vi "extract_value_from_string.vi"(8 "error in (no error)":errorcluster, 11 "Input string":string) -> (0 "error out":errorcluster, 2 "Value":dbl, 3 "Rest of string":string)   [LabVIEW 2016, in "Chemyx_Syringe_Pump_driver.lvlib"]
doc: "Converts the first number of an input string into a number and output the rest of the string."
uses:
  Chemyx_Syringe_Pump_driver.lvlib
panel:
  # "Converts the first number of an input string into a number and output the rest of the string."
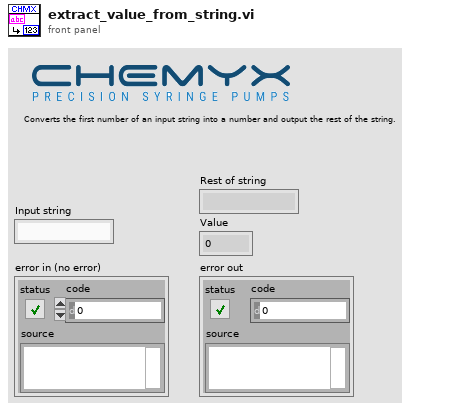
[diagram p1: front panel]
types:
  T1 = enum16{"Native", "Native Command Line", "UNIX", "Macintosh", "DOS"}
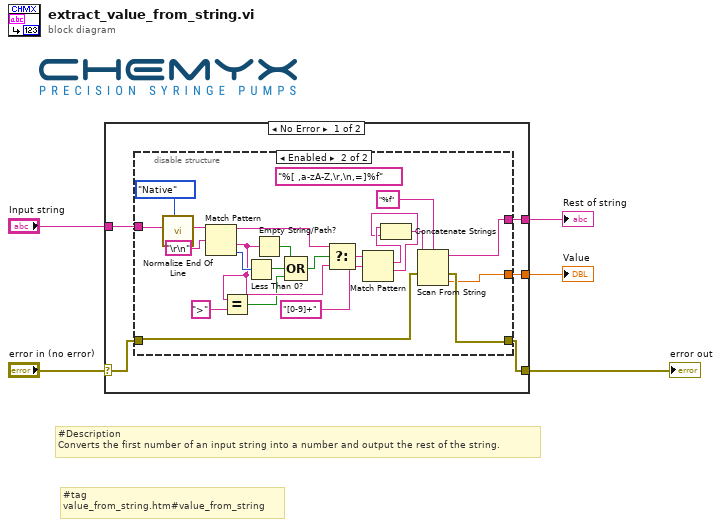
[diagram p0: block diagram]
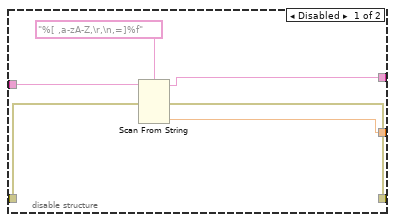
[diagram p2: hidden frame]
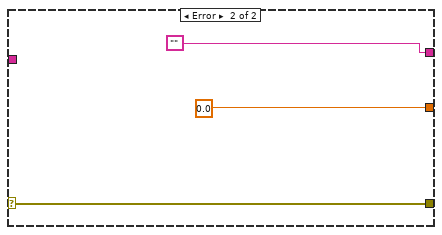
[diagram p3: hidden frame]
diagram:
  # "#tag\nvalue_from_string.htm#value_from_string"
  # "#Description\nConverts the first number of an input string into a number and output the rest of the string."
  n1 = case shown="No Error" "error in (no error)" {
    selector: "error in (no error)" -> [w10 w39]
    tunnel: [w9 w39] -> w4
    tunnel: "Input string" -> [w8 _]
    tunnel: [w7 0.0] -> w2
    tunnel: [w6 ""] -> w1
    frame No Error {
      n2 = disable-structure shown="Enabled" {
        disable-tunnel: w10 -> [w16 w27]
        disable-tunnel: [w14 w26] -> w9
        disable-tunnel: w8 -> [w13 w38]
        disable-tunnel: [w12 w20] -> w7
        disable-tunnel: [w11 w28] -> w6
        frame Disabled {
          n3 = Scan From String(format string="%[ ,a-zA-Z,\r,\n,=]%f", input string=w13, error in=w16) -> (remaining string=w11:string, error out=w14:errorcluster, output 2=w12:dbl)  [unwired: 4 in, 1 out]
        }
        frame Enabled {
          (unwired) "%[ ,a-zA-Z,\r,\n,=]%f" ("format string")
          n4 = call <vilib>:"Normalize End Of Line.vi"("end of line (Native)"=T1."Native", "string in"=w38) -> ("string out"=w36:string)  [unwired: 6 in]
          n5 = Match Pattern(string=w36, regular expression="\r\n") -> (before substring=w30:string, after substring=w19:string, offset past match=w34:i32)  [unwired: 1 in, 1 out]
          n6 = Equal?(x=w19, y=">") -> (x = y?=w17:bool)
          n7 = Less Than 0?(x=w34) -> (x < 0?=w33:bool)
          n8 = Empty String/Path?(string/path=w19) -> (empty?=w32:bool)
          n9 = Compound Arithmetic op=OR(w32, w33, w17) -> (w31:bool)
          n10 = Select(t=w30, s=w31, f=w19) -> (s? t:f=w25:string)
          n11 = Match Pattern(string=w25, regular expression="[0-9]+") -> (match substring=w23:string, after substring=w22:string)  [unwired: 1 in, 2 out]
          n12 = Concatenate Strings(w23, w22) -> (w21:string)
          n13 = Scan From String(format string="%f", input string=w21, error in=w27) -> (remaining string=w28:string, error out=w26:errorcluster, output 1=w20:dbl)  [unwired: 2 in, 1 out]
        }
      }
    }
    frame Error {
    }
  }
  "error out" <- w4
  "Value" <- w2
  "Rest of string" <- w1
